vi "DSF.Shared.Configuration.Set ID.vi"(10 "id":T1, 11 "Configuration in":refnum<class "DSF.Shared.Configuration.lvclass">) -> (3 "Configuration out":refnum<class "DSF.Shared.Configuration.lvclass">)   [LabVIEW 2016, in "DSF.Shared.lvlib" / "DSF.Shared.Configuration.lvclass"]
uses:
  DSF.Shared.Configuration.lvclass
  Typedefs/DSF.Shared.Typedefs.ID.ctl
  DSF.Shared.Configuration.lvclass/DSF.Shared.Configuration.ctl
  DSF.Shared.lvlib
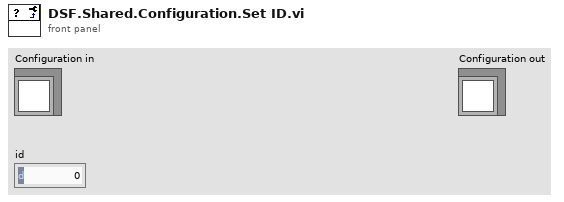
[diagram p1: front panel]
types:
  T1 = typedef "DSF.Shared.lvlib/DSF.Shared.Typedefs.ID.ctl" = i32
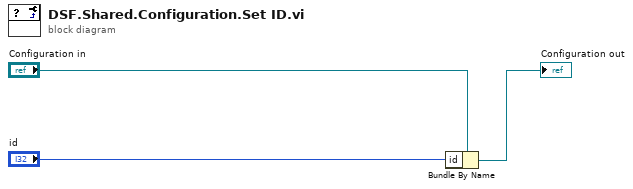
[diagram p0: block diagram]
diagram:
  n1 = Bundle By Name(cluster="Configuration in", "id"="id") -> (→"Configuration out":refnum<class "DSF.Shared.Configuration.lvclass">)
